vi "gl_X-Grapher refs.vi"() -> ()   [LabVIEW 2020]
uses:
  Typedefs/Xctrl-Waveform graph ref.ctl
  Typedefs/Xctrl-Timeline graph ref.ctl
  XGrapher.xctl
panel:
  out "X-Grapher refs":cluster{"XY Graph":T1, "Timeline Graph":T2}
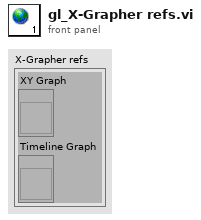
[diagram p1: front panel]
types:
  T1 = typedef "XGrapher.xctl/Xctrl-Waveform graph ref.ctl" = refnum<vi>
  T2 = typedef "XGrapher.xctl/Xctrl-Timeline graph ref.ctl" = refnum<vi>
diagram:
